vi "Measuring Complete Example (A).vi"() -> ()   [LabVIEW 2011]
uses:
  C:/Program Files/Metrohm Autolab/Autolab SDK 1.10/EcoChemie.Autolab.Sdk.dll
  EcoChemie.Autolab.Sdk.dll
panel:
  out "PotentialApplied":dbl
  in  "Abort":bool
  in  "fileName":string
  out "IsMeasuring":bool
  in  "Save":bool
  in  "start measure":bool
  out "Value Y":dbl
  out "Value X":dbl
  out "XY Graph 2":cluster{"Y":dbl[], "Y":dbl[]}[](graph)
  in  "Signal X":string(combo)
  in  "Signal Y":string(combo)
  in  "Embedded Exe File":path
  out "Contains blacklist item":bool
  out "0, 1":i16
  in  "BoolSet":bool
  out "GetSetDoubleValue":dbl
  out "EnumGet":i32(ring) items=["Off", "On"]
  in  "SetEnum":bool
  in  "EnumSet":i32(ring) items=["Off", "On"]
  in  "Command":string(combo)
  in  "Command Parameter":string(combo)
  out "DoubleGet":dbl
  out "IntGet":i32
  in  "DoubleSet":dbl
  in  "IntSet":i32
  in  "SetBool":bool
  in  "SetDouble":bool
  in  "SetInt":bool
  in  "GetSet Parameter":bool
  in  "Hardware Setup File":path
  in  "Load":bool
  in  "data":bool
  out "error out":errorcluster
  in  "Stop":bool
  in  "Signal Y":string(combo)
  in  "Signal X":string(combo)
  in  "ProcedureCommandList":string(combo)
  out "XY Graph":cluster{"Values":dbl[], "Values":dbl[]}(graph)
  out "Value Y":dbl[](array[numeric])
  out "Value X":dbl[](array[numeric])
  in  "Procedure":path=path "Standard Nova Procedures/Chrono amperometry.nox"
  out "IsConnected":bool
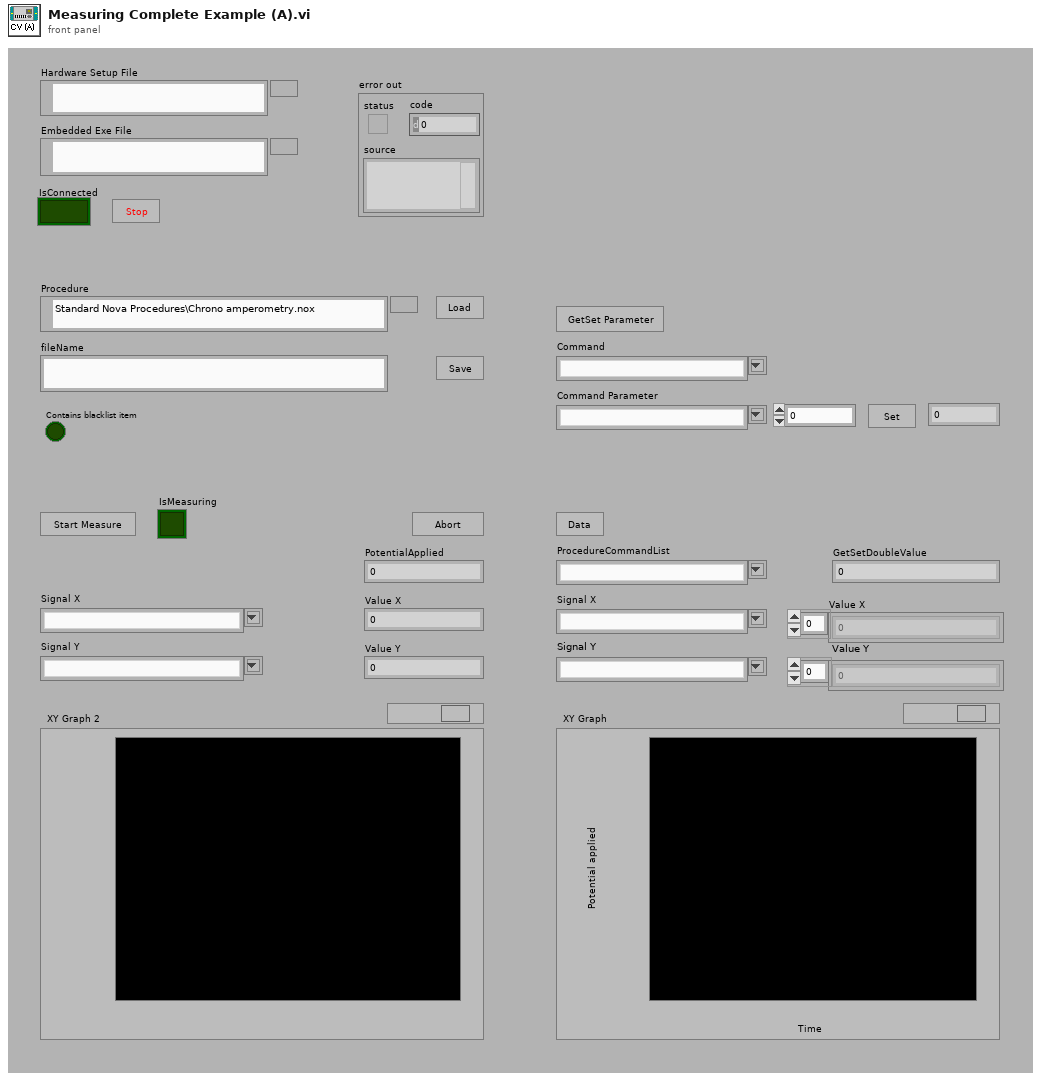
[diagram p1: front panel]
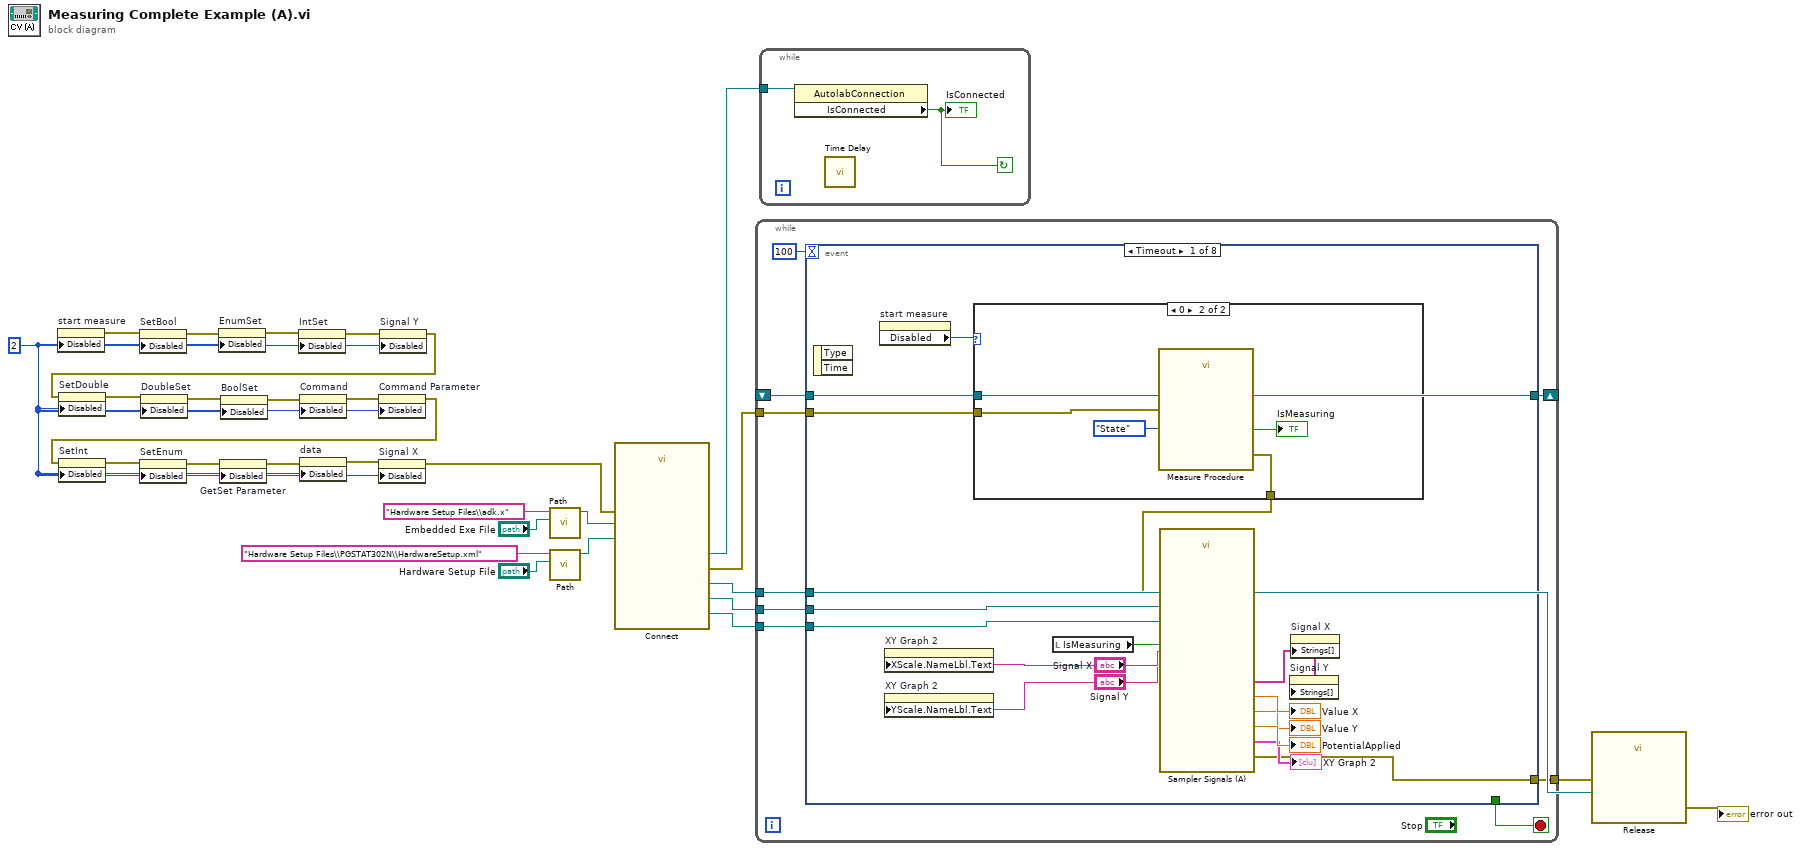
[diagram p0: block diagram]
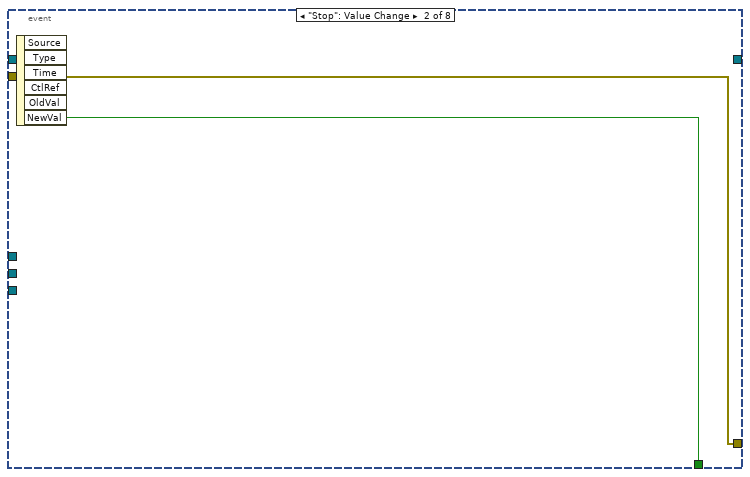
[diagram p3: hidden frame]
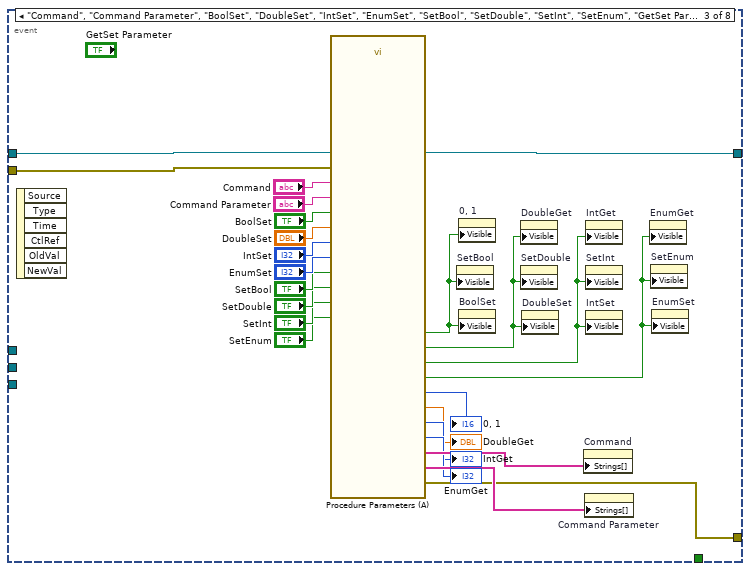
[diagram p4: hidden frame]
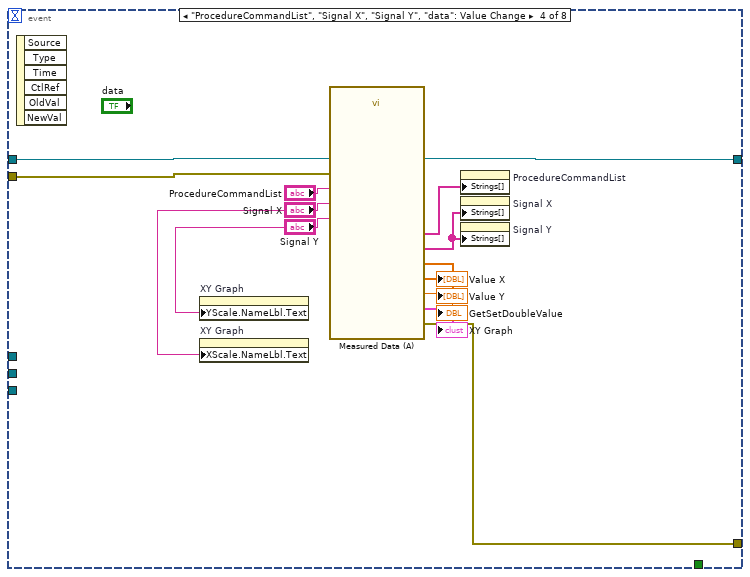
[diagram p5: hidden frame]
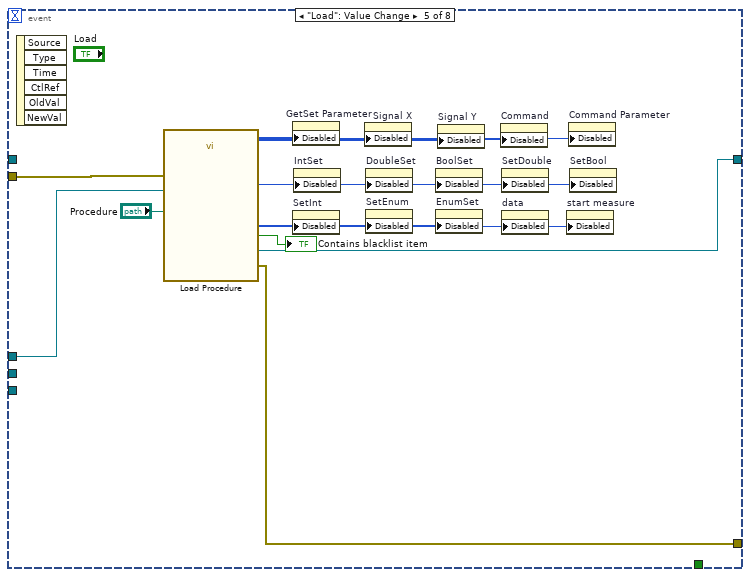
[diagram p6: hidden frame]
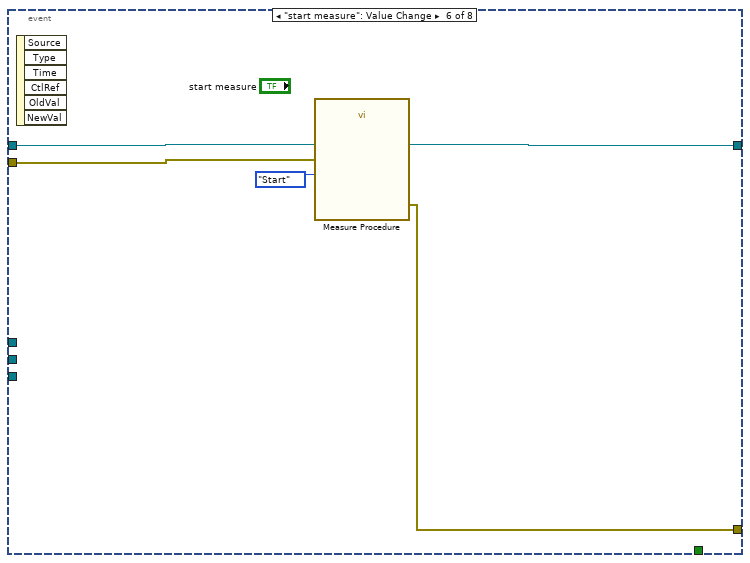
[diagram p7: hidden frame]
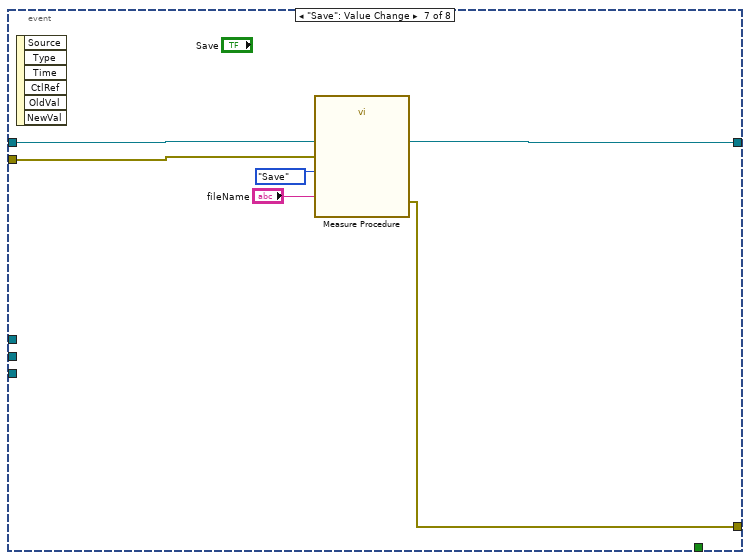
[diagram p8: hidden frame]
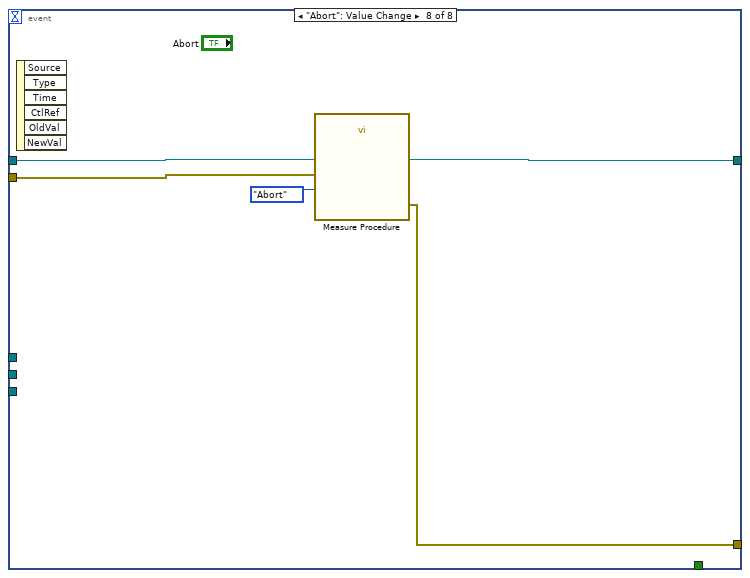
[diagram p9: hidden frame]
diagram:
  w9 = u8 2 ("Disabled")
  n1 = property on="start measure" class="Bool"("Disabled"=w9) -> (error out=w14:errorcluster)  [unwired: 2 in, 1 out]
  n2 = property on="SetBool" class="Bool (strict)"(error in=w14, "Disabled"=w9) -> (error out=w24:errorcluster)  [unwired: 1 in, 1 out]
  n3 = property on="EnumSet" class="Ring (strict)"(error in=w24, "Disabled"=w9) -> (error out=w23:errorcluster)  [unwired: 1 in, 1 out]
  n4 = property on="IntSet" class="DigNum (strict)"(error in=w23, "Disabled"=w9) -> (error out=w22:errorcluster)  [unwired: 1 in, 1 out]
  n5 = property on="Signal Y" class="CmbBox"(error in=w22, "Disabled"=w9) -> (error out=w13:errorcluster)  [unwired: 1 in, 1 out]
  n6 = property on="SetDouble" class="Bool (strict)"(error in=w13, "Disabled"=w9) -> (error out=w12:errorcluster)  [unwired: 1 in, 1 out]
  n7 = property on="DoubleSet" class="DigNum (strict)"(error in=w12, "Disabled"=w9) -> (error out=w21:errorcluster)  [unwired: 1 in, 1 out]
  n8 = property on="BoolSet" class="Bool (strict)"(error in=w21, "Disabled"=w9) -> (error out=w20:errorcluster)  [unwired: 1 in, 1 out]
  n9 = property on="Command" class="CmbBox"(error in=w20, "Disabled"=w9) -> (error out=w19:errorcluster)  [unwired: 1 in, 1 out]
  n10 = property on="Command Parameter" class="CmbBox"(error in=w19, "Disabled"=w9) -> (error out=w11:errorcluster)  [unwired: 1 in, 1 out]
  n11 = property on="SetInt" class="Bool (strict)"(error in=w11, "Disabled"=w9) -> (error out=w10:errorcluster)  [unwired: 1 in, 1 out]
  n12 = property on="SetEnum" class="Bool (strict)"(error in=w10, "Disabled"=w9) -> (error out=w18:errorcluster)  [unwired: 1 in, 1 out]
  n13 = property on="GetSet Parameter" class="Bool (strict)"(error in=w18, "Disabled"=w9) -> (error out=w17:errorcluster)  [unwired: 1 in, 1 out]
  n14 = property on="data" class="Bool"(error in=w17, "Disabled"=w9) -> (error out=w16:errorcluster)  [unwired: 1 in, 1 out]
  n15 = property on="Signal X" class="CmbBox"(error in=w16, "Disabled"=w9) -> (error out=w15:errorcluster)  [unwired: 1 in, 1 out]
  n16 = call "Path.vi"("File"="Embedded Exe File", "name or relative path"="Hardware Setup Files\\adk.x") -> ("appended path"=w4:path)  [unwired: 9 in]
  n17 = call "Path.vi"("File"="Hardware Setup File", "name or relative path"="Hardware Setup Files\\PGSTAT302N\\HardwareSetup.xml") -> ("appended path"=w3:path)  [unwired: 9 in]
  n18 = call "Connect.vi"("Embedded Exe File"=w4, "Hardware Setup File"=w3, "error in (no error)"=w15) -> ("Sampler"=w26:refnum<k24>, "AutolabConnection"=w28:refnum<k24>, "instrument"=w7:refnum<k24>, "Ei"=w27:refnum<k24>, "error out"=w25:errorcluster)  [unwired: 5 in, 3 out]
  n19 = while {
    tunnel: w27 -> [w37]
    tunnel: w26 -> [w36]
    shift-right: [w35] -> _
    shift-left: _ -> [w34]
    tunnel: w25 -> [w33]
    tunnel: w7 -> [w32]
    tunnel: [w30] -> w8
    stop <- w38 stop-if-true
    n20 = event shown="[0] Timeout" {
      selector: _ -> [_ _ _ _ _ _ _ _]
      dyn-events: _ -> [_ _ _ _ _ _ _ _]
      timeout: 100 -> [_ _ _ _ _ _ _ _]
      tunnel: [_ w61 _ _ _ _ _ _] -> w38
      tunnel: w37 -> [w44 _ _ _ _ _ _ _]
      tunnel: w36 -> [w43 _ _ _ _ _ _ _]
      tunnel: [w41 _ w64 w87 w101 w107 w112 w116] -> w35
      tunnel: w34 -> [w41 _ w64 w87 _ w107 w112 w116]
      tunnel: w33 -> [w40 w60 w63 w86 w100 w106 w111 w115]
      tunnel: w32 -> [_ _ _ _ w99 _ _ _]
      tunnel: [w39 w60 w62 w85 w98 w104 w110 w113] -> w30
      event Timeout {
        n21 = event-data() -> ()  [unwired: 1 in, 2 out]
        n22 = property on="start measure" class="Bool"() -> ("Disabled"=w45:u8)  [unwired: 2 in, 2 out]
        n23 = property on="XY Graph 2" class="XYGraph (strict)"("XScale.NameLbl.Text"="Signal X") -> ()  [unwired: 2 in, 2 out]
        n24 = property on="XY Graph 2" class="XYGraph (strict)"("YScale.NameLbl.Text"="Signal Y") -> ()  [unwired: 2 in, 2 out]
        n25 = case shown="0" w45 {
          tunnel: [w54 w57] -> w42
          tunnel: w41 -> [_ w56]
          tunnel: w40 -> [w54 w55]
          frame 2, Default {
          }
          frame 0 {
            n26 = call "Measure Procedure.vi"("error in"=w55, "Request for procedure"=enum16{"State", "Save", "Abort", "Start"}."State", "LoadProcedure"=w56) -> ("error out"=w57:errorcluster, "IsMeasuring"=→"IsMeasuring":bool)  [unwired: 7 in]
          }
        }
        n27 = local read "IsMeasuring"() -> (w52:bool)
        n28 = call "Sampler Signals (A).vi"("IsMeasuring"=w52, "EI"=w44, "Sampler"=w43, "Signal X"="Signal X", "Signal Y"="Signal Y", "error in"=w42) -> ("PotentialApplied"=→"PotentialApplied":dbl, "X"=→"Value X":dbl, "Y"=→"Value Y":dbl, "XY Graph"=→"XY Graph 2":cluster{"Y":dbl[], "Y":dbl[]}[], "GetSignals"=w49:string[], "error out"=w39:errorcluster)  [unwired: 4 in]
        n29 = property on="Signal Y" class="CmbBox"("Strings[]"=w49) -> ()  [unwired: 2 in, 2 out]
        n30 = property on="Signal X" class="CmbBox"("Strings[]"=w49) -> ()  [unwired: 2 in, 2 out]
      }
      event "Stop": Value Change {
        n31 = event-data() -> ("NewVal"=w61:bool)  [unwired: 1 in, 5 out]
      }
      event "Command", "Command Parameter", "BoolSet", "DoubleSet", "IntSet", "EnumSet", "SetBool", "SetDouble", "SetInt", "SetEnum", "GetSet Parameter": Value Change {
        n32 = event-data() -> ()  [unwired: 1 in, 6 out]
        n33 = call "Procedure Parameters (A).vi"("LoadProcedure"=w64, "Command"="Command", "Command Parameter"="Command Parameter", "EnumSet"="EnumSet", "DoubleSet"="DoubleSet", "IntSet"="IntSet", "BoolSet"="BoolSet", "SetEnum"="SetEnum", "SetDouble"="SetDouble", "SetInt"="SetInt", "SetBool"="SetBool", "error in (no error)"=w63) -> ("error out"=w62:errorcluster, "IntGet"=→"IntGet":i32, "0, 1"=→"0, 1":i16, "EnumGet"=→"EnumGet":i32, "DoubleGet"=→"DoubleGet":dbl, "Command Names"=w83:string[], "Command Parameters"=w84:string[], "VisibleEnum"=w78:bool, "VisibleInt"=w77:bool, "VisibleDouble"=w76:bool, "VisableBool"=w75:bool)  [unwired: 5 in]
        n34 = property on="SetBool" class="Bool (strict)"("Visible"=w75) -> ()  [unwired: 2 in, 2 out]
        n35 = property on="0, 1" class="DigNum (strict)"("Visible"=w75) -> ()  [unwired: 2 in, 2 out]
        n36 = property on="BoolSet" class="Bool (strict)"("Visible"=w75) -> ()  [unwired: 2 in, 2 out]
        n37 = property on="DoubleGet" class="DigNum (strict)"("Visible"=w76) -> ()  [unwired: 2 in, 2 out]
        n38 = property on="SetDouble" class="Bool (strict)"("Visible"=w76) -> ()  [unwired: 2 in, 2 out]
        n39 = property on="DoubleSet" class="DigNum (strict)"("Visible"=w76) -> ()  [unwired: 2 in, 2 out]
        n40 = property on="Command" class="CmbBox"("Strings[]"=w83) -> ()  [unwired: 2 in, 2 out]
        n41 = property on="Command Parameter" class="CmbBox"("Strings[]"=w84) -> ()  [unwired: 2 in, 2 out]
        n42 = property on="IntGet" class="DigNum (strict)"("Visible"=w77) -> ()  [unwired: 2 in, 2 out]
        n43 = property on="SetInt" class="Bool (strict)"("Visible"=w77) -> ()  [unwired: 2 in, 2 out]
        n44 = property on="IntSet" class="DigNum (strict)"("Visible"=w77) -> ()  [unwired: 2 in, 2 out]
        n45 = property on="EnumGet" class="Ring (strict)"("Visible"=w78) -> ()  [unwired: 2 in, 2 out]
        n46 = property on="SetEnum" class="Bool (strict)"("Visible"=w78) -> ()  [unwired: 2 in, 2 out]
        n47 = property on="EnumSet" class="Ring (strict)"("Visible"=w78) -> ()  [unwired: 2 in, 2 out]
      }
      event "ProcedureCommandList", "Signal X", "Signal Y", "data": Value Change {
        n48 = event-data() -> ()  [unwired: 1 in, 6 out]
        n49 = property on="XY Graph" class="XYGraph (strict)"("YScale.NameLbl.Text"="Signal Y") -> ()  [unwired: 2 in, 2 out]
        n50 = property on="XY Graph" class="XYGraph (strict)"("XScale.NameLbl.Text"="Signal X") -> ()  [unwired: 2 in, 2 out]
        n51 = call "Measured Data (A).vi"("LoadProcedure"=w87, "ProcedureCommandList"="ProcedureCommandList", "Signal X sel"="Signal X", "Signal Y sel"="Signal Y", "error in (no error)"=w86) -> ("Value Y"=→"Value Y":dbl[], "Signal Names"=w90:string[], "ProcedureCommandList"=w89:string[], "Value"=→"GetSetDoubleValue":dbl, "Value X"=→"Value X":dbl[], "XY Graph"=→"XY Graph":cluster{"Values":dbl[], "Values":dbl[]}, "error out"=w85:errorcluster)  [unwired: 4 in]
        n52 = property on="ProcedureCommandList" class="CmbBox"("Strings[]"=w89) -> ()  [unwired: 2 in, 2 out]
        n53 = property on="Signal X" class="CmbBox"("Strings[]"=w90) -> ()  [unwired: 2 in, 2 out]
        n54 = property on="Signal Y" class="CmbBox"("Strings[]"=w90) -> ()  [unwired: 2 in, 2 out]
      }
      event "Load": Value Change {
        n55 = event-data() -> ()  [unwired: 1 in, 6 out]
        n56 = call "Load Procedure.vi"("error in (no error)"=w100, "Procedure"="Procedure", "Instrument"=w99) -> ("error out"=w98:errorcluster, "Contains"=→"Contains blacklist item":bool, "Numeric"=w97:i32, "LoadProcedure"=w101:refnum<k24>)  [unwired: 5 in]
        n57 = property on="GetSet Parameter" class="Bool (strict)"("Disabled"=w97) -> ()  [unwired: 2 in, 2 out]
        n58 = property on="SetInt" class="Bool (strict)"("Disabled"=w97) -> ()  [unwired: 2 in, 2 out]
        n59 = property on="IntSet" class="DigNum (strict)"("Disabled"=w97) -> ()  [unwired: 2 in, 2 out]
        n60 = property on="Signal X" class="CmbBox"("Disabled"=w97) -> ()  [unwired: 2 in, 2 out]
        n61 = property on="DoubleSet" class="DigNum (strict)"("Disabled"=w97) -> ()  [unwired: 2 in, 2 out]
        n62 = property on="SetEnum" class="Bool (strict)"("Disabled"=w97) -> ()  [unwired: 2 in, 2 out]
        n63 = property on="BoolSet" class="Bool (strict)"("Disabled"=w97) -> ()  [unwired: 2 in, 2 out]
        n64 = property on="EnumSet" class="Ring (strict)"("Disabled"=w97) -> ()  [unwired: 2 in, 2 out]
        n65 = property on="Signal Y" class="CmbBox"("Disabled"=w97) -> ()  [unwired: 2 in, 2 out]
        n66 = property on="Command" class="CmbBox"("Disabled"=w97) -> ()  [unwired: 2 in, 2 out]
        n67 = property on="SetDouble" class="Bool (strict)"("Disabled"=w97) -> ()  [unwired: 2 in, 2 out]
        n68 = property on="data" class="Bool"("Disabled"=w97) -> ()  [unwired: 2 in, 2 out]
        n69 = property on="start measure" class="Bool"("Disabled"=w97) -> ()  [unwired: 2 in, 2 out]
        n70 = property on="Command Parameter" class="CmbBox"("Disabled"=w97) -> ()  [unwired: 2 in, 2 out]
        n71 = property on="SetBool" class="Bool (strict)"("Disabled"=w97) -> ()  [unwired: 2 in, 2 out]
      }
      event "start measure": Value Change {
        n72 = event-data() -> ()  [unwired: 1 in, 6 out]
        n73 = call "Measure Procedure.vi"("error in"=w106, "Request for procedure"=enum16{"State", "Save", "Abort", "Start"}."Start", "LoadProcedure"=w107) -> ("error out"=w104:errorcluster)  [unwired: 7 in, 1 out]
      }
      event "Save": Value Change {
        n74 = event-data() -> ()  [unwired: 1 in, 6 out]
        n75 = call "Measure Procedure.vi"("error in"=w111, "fileName"="fileName", "Request for procedure"=enum16{"State", "Save", "Abort", "Start"}."Save", "LoadProcedure"=w112) -> ("error out"=w110:errorcluster)  [unwired: 6 in, 1 out]
      }
      event "Abort": Value Change {
        n76 = event-data() -> ()  [unwired: 1 in, 6 out]
        n77 = call "Measure Procedure.vi"("error in"=w115, "Request for procedure"=enum16{"State", "Save", "Abort", "Start"}."Abort", "LoadProcedure"=w116) -> ("error out"=w113:errorcluster)  [unwired: 7 in, 1 out]
      }
    }
  }
  n78 = while {
    tunnel: w28 -> [w117]
    stop <- w118 continue-if-true
    n79 = property class="AutolabConnection"(reference=w117) -> ("IsConnected"=w118:bool)  [unwired: 1 in, 2 out]
    "IsConnected" <- w118
    n80 = call "Time Delay"() -> ()  [unwired: 11 in, 1 out]
  }
  n81 = call "Release.vi"("error in (no error)"=w8, "Instrument"=w7) -> ("error out"=→"error out":errorcluster)  [unwired: 9 in]
